vi "Remove Correction Table Entries.vi"(7 "Interval End (24e6)":dbl=24000000.0 format="%^.3e", 8 "error in (no error)":errorcluster, 9 "Interval Start (24e6)":dbl=24000000.0 format="%^.3e", 10 "Correction Table (\"Table1\")":string="Table1", 11 "VISA resource name":refnum<visa-resource-name>) -> (0 "error out":errorcluster, 3 "VISA resource name out":refnum<visa-resource-name>)   [LabVIEW 2020, in "Rohde&Schwarz CMXP Base.lvlib"]
doc: "Removes entries from an existing correction table.\n\nTo remove all entries in a certain frequency range, enter the lower frequency as Interval Start and the upper frequency as Interval End.\n\nAttribute:\n-\n\nRemote-control command:\nREMove:SYSTem:ATTenuation:CTABle"
uses:
  <instrlib>/Rohde&Schwarz CMXP Base/Rohde&Schwarz CMXP Base.lvlib
  <instrlib>/Rohde&Schwarz CMXP Base/Private/rsidr_core.llb/rsidr_core.lvlib
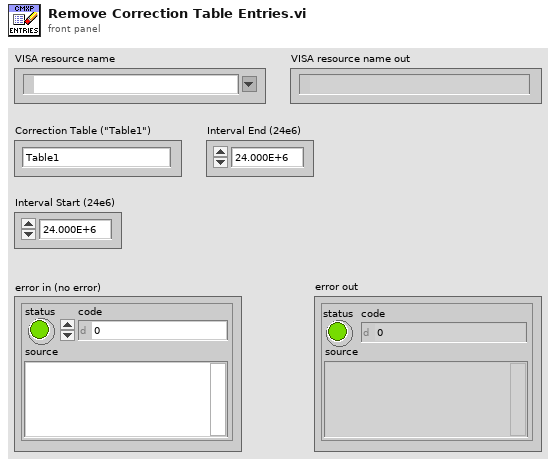
[diagram p1: front panel]
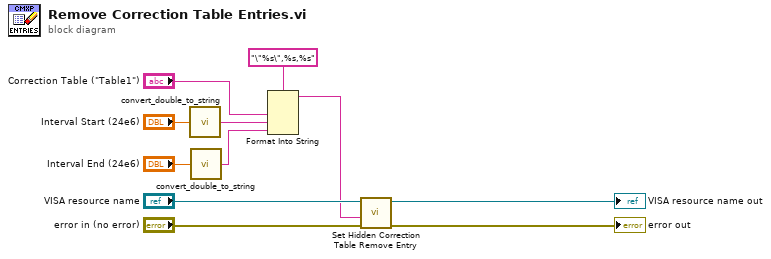
[diagram p0: block diagram]
diagram:
  n1 = call <instrlib>:"convert_double_to_string.vi"("double in"="Interval Start (24e6)") -> ("string out"=w3:string)  [unwired: 4 in]
  n2 = call <instrlib>:"convert_double_to_string.vi"("double in"="Interval End (24e6)") -> ("string out"=w2:string)  [unwired: 4 in]
  n3 = Format Into String(format string="\"%s\",%s,%s", "Correction Table (\"Table1\")", w3, w2) -> (resulting string=w1:string)  [unwired: 2 in, 1 out]
  n4 = call "Set Hidden Correction Table Remove Entry"("error in (no error)"="error in (no error)", "Hidden Correction Table Remove Entry ()"=w1, "instrument handle"="VISA resource name") -> ("error out"=→"error out":errorcluster, "instrument handle out"=→"VISA resource name out":refnum<visa-resource-name>)  [unwired: 7 in]
